vi "run.vi"(8 "error in (no error)":errorcluster, 11 "GenericDAQ in":refnum<class "GenericDAQ.lvclass">) -> (0 "error out":errorcluster, 3 "GenericDAQ out":refnum<class "GenericDAQ.lvclass">)   [LabVIEW 2010, in "GenericDAQ.lvclass"]
uses:
  GenericDAQ.lvclass
  common/classes/ErrorController/ErrorController/class_data.vi
  common/classes/ErrorController/ErrorController/ErrorController.lvclass
panel:
  in  "Tab Control":enum32{"User", "Debug", "About"}(tab)
  out "trigger loop counter":i32
  # "This is a dummy component with no functionality."
  # "GenericDAQ\n\nImplemented by: \n- Dominik Langer, University of Zurich, Switzerland"
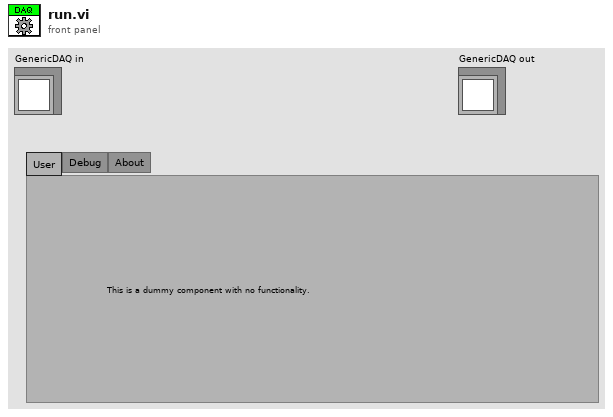
[diagram p1: front panel]
types:
  T1 = typedef "main_trigger_enum.ctl" = enum16{"NULL", "initialise", "terminate", "start", "stop", "change objective", "change experimentController", "change imagingMode", "save notebook", "started saving", "finished saving", "expCtr ready", "expCtr missing", "imgMd ready", "imgMd missing", "scanHd ready", "scanHd missing", "DAQ ready", "DAQ missing", "imgAsm ready", "imgAsm missing", "dataColl ready", "dataColl missing", "display ready", "display missing", "analysr ready", "analysr missing", "instrmnt ready", "instrmnt missing", "stimltr ready", "stimltr missing", "stage ready", "stage missing"}
  T2 = typedef "GenericToplevelComponent.lvclass/common_trigger_enum.ctl" = enum16{"NULL", "initialise", "terminate", "fetch command", "fetch data", "attach observer", "register as observer", "detach observer", "acknowledge", "start", "stop", "sweep started", "sweep finished", "experiment started", "experiment stopped"}
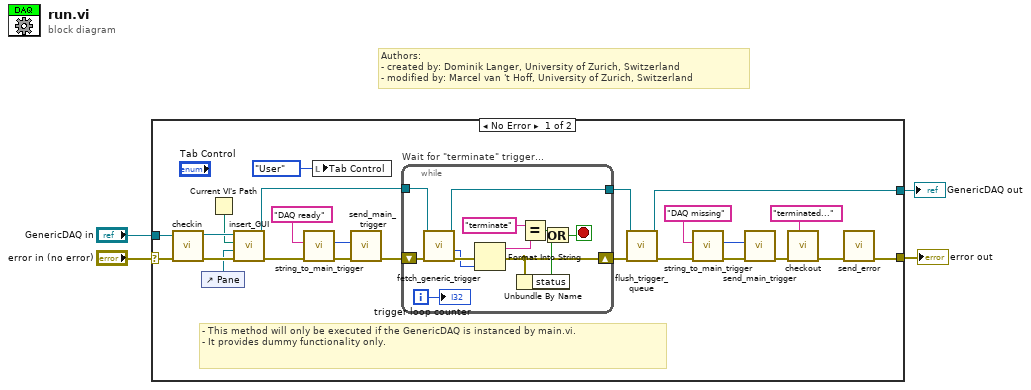
[diagram p0: block diagram]
diagram:
  # "Authors: \n- created by: Dominik Langer, University of Zurich, Switzerland\n- modified by: Marcel van 't Hoff, University of Zurich, Switzerland"
  n1 = case shown="No Error" "error in (no error)" {
    selector: "error in (no error)" -> [w28 w42]
    tunnel: [w18 w42] -> w3
    tunnel: [w15 w41] -> w1
    tunnel: "GenericDAQ in" -> [w27 w41]
    frame No Error {
      # "- This method will only be executed if the GenericDAQ is instanced by main.vi.\n- It provides dummy functionality only."
      n2 = call-dynamic "checkin.vi"("error in (no error)"=w28, "GenericDAQ in"=w27) -> ("error out"=w23:errorcluster, "GenericDAQ out"=w24:refnum<class "GenericDAQ.lvclass">)  [unwired: 8 in]
      n3 = control-ref of="Pane"() -> (w20:refnum<vi>)
      n4 = Current VI's Path() -> (path=w22:path)
      n5 = call-dynamic "insert_GUI.vi"("error in (no error)"=w23, "Pane"=w20, "VI path"=w22, "GenericComponent in"=w24) -> ("error out"=w8:errorcluster, "GenericComponent out"=w16:refnum<class "GenericDAQ.lvclass">)  [unwired: 6 in]
      n6 = call "string_to_main_trigger.vi"("error in (no error)"=w8, "trigger string"="DAQ ready" ("input string")) -> ("error out"=w7:errorcluster, "main trigger"=w5:T1)  [unwired: 8 in]
      n7 = local write "Tab Control"(enum32{"User", "Debug", "About"}."User" ("Tab Control")) -> ()
      n8 = call "send_main_trigger.vi"("error in (no error)"=w7, "trigger"=w5) -> ("error out"=w25:errorcluster)  [unwired: 9 in]
      n9 = while "Wait for \"terminate\" trigger..." {
        tunnel: w16 -> [w35]
        tunnel: [w34] -> w13
        shift-right: [w33] -> w17
        shift-left: w25 -> [w36]
        i -> [w40]
        stop <- w37 stop-if-true
        n10 = call-dynamic "fetch_generic_trigger.vi"("error in (no error)"=w36, "GenericToplevelComponent in"=w35) -> ("error out"=w32:errorcluster, "common trigger"=w31:T2, "GenericToplevelComponent out"=w34:refnum<class "GenericDAQ.lvclass">)  [unwired: 3 in, 4 out]
        n11 = Format Into String(error in=w32, w31) -> (resulting string=w30:string, error out=w33:errorcluster)  [unwired: 2 in]
        n12 = Unbundle By Name(w33) -> ("status"=w38:bool)
        n13 = Equal?(x="terminate", y=w30) -> (x = y?=w39:bool)
        n14 = Or(x=w39, y=w38) -> (x .or. y?=w37:bool)
        "trigger loop counter" <- w40
      }
      n15 = call-dynamic "flush_trigger_queue.vi"("error in (no error)"=w17, "GenericToplevelComponent in"=w13) -> ("error out"=w12:errorcluster, "GenericToplevelComponent out"=w15:refnum<class "GenericDAQ.lvclass">)  [unwired: 8 in]
      n16 = call "string_to_main_trigger.vi"("error in (no error)"=w12, "trigger string"="DAQ missing" ("input string")) -> ("error out"=w11:errorcluster, "main trigger"=w10:T1)  [unwired: 8 in]
      n17 = call "send_main_trigger.vi"("error in (no error)"=w11, "trigger"=w10) -> ("error out"=w26:errorcluster)  [unwired: 9 in]
      n18 = call "checkout.vi"("locked by?"="terminated...", "error in (no error)"=w26) -> ("error out"=w19:errorcluster)  [unwired: 8 in, 1 out]
      n19 = call "send_error.vi"("error in (no error)"=w19) -> ("error out"=w18:errorcluster)  [unwired: 10 in]
    }
    frame Error {
    }
  }
  "error out" <- w3
  "GenericDAQ out" <- w1
